vi "Receive Value Change Event.vi"(8 "error in (no error)":errorcluster, 10 "ValueChangeMsg":refnum<class "ValueChangeMsg.lvclass">, 11 "For Loop Dialog In":refnum<class "Conditional Dialog.lvclass">) -> (0 "error out":errorcluster, 3 "For Loop Dialog Out":refnum<class "Conditional Dialog.lvclass">)   [LabVIEW 2017, in "Conditional Dialog.lvclass"]
doc: "<License>\nCopyright © 2017 Composed Systems, LLC | All rights reserved\nwww.composed.io\n\nAuthor: Ethan Stern <ethan.stern@composed.io>\n\nThis software is provided \"AS IS\" WITHOUT WARRANTIES, either express or implied, AND IS FOR EDUCATIONAL PURPOSES ONLY.\n</License>"
uses:
  Conditional Dialog.lvclass
  ITest Executive Builder Dialog/ITest Executive Builder Dialog.lvclass
  <vilib>/gpm_packages/@cs/mva-viewable/Source/ActorEvents/IEventAggregator Messages/ValueChangeMsg/ValueChangeMsg.lvclass
  <vilib>/ActorFramework/Actor/Actor.lvclass
  <vilib>/ActorFramework/Stop Msg/Stop Msg.lvclass
  698eee39-0e44-4932-ada2-d875f71f8c5a.vi
  C:/Program Files (x86)/National Instruments/LabVIEW 2017/vi.lib/ActorFramework/Actor/Actor.lvclass
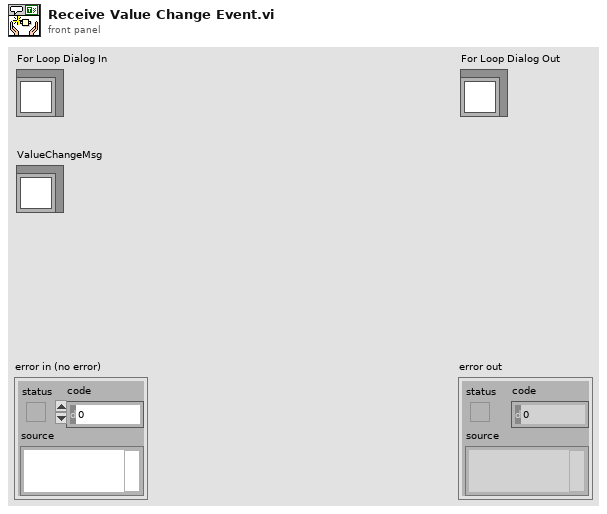
[diagram p1: front panel]
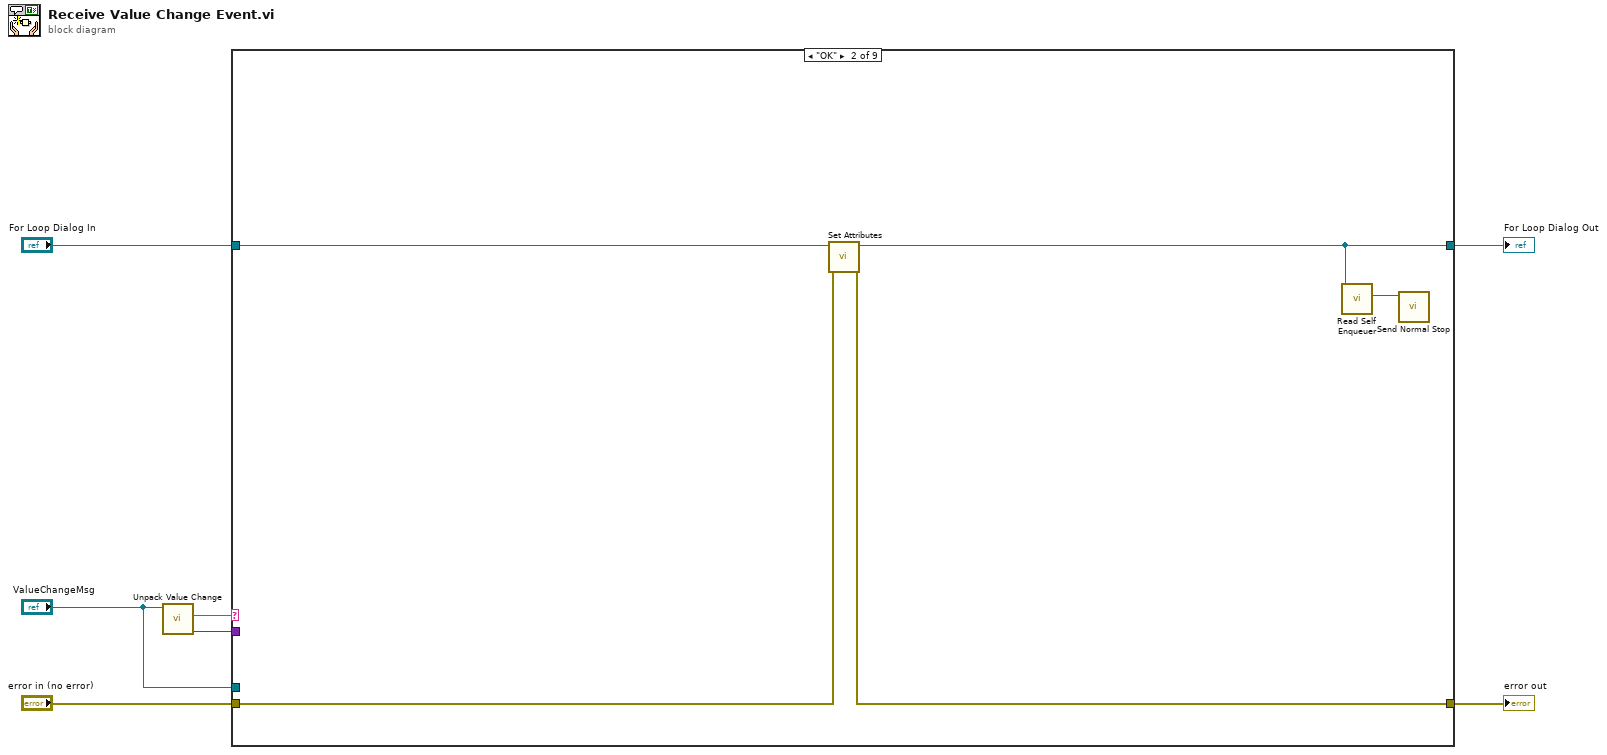
[diagram p0: block diagram]
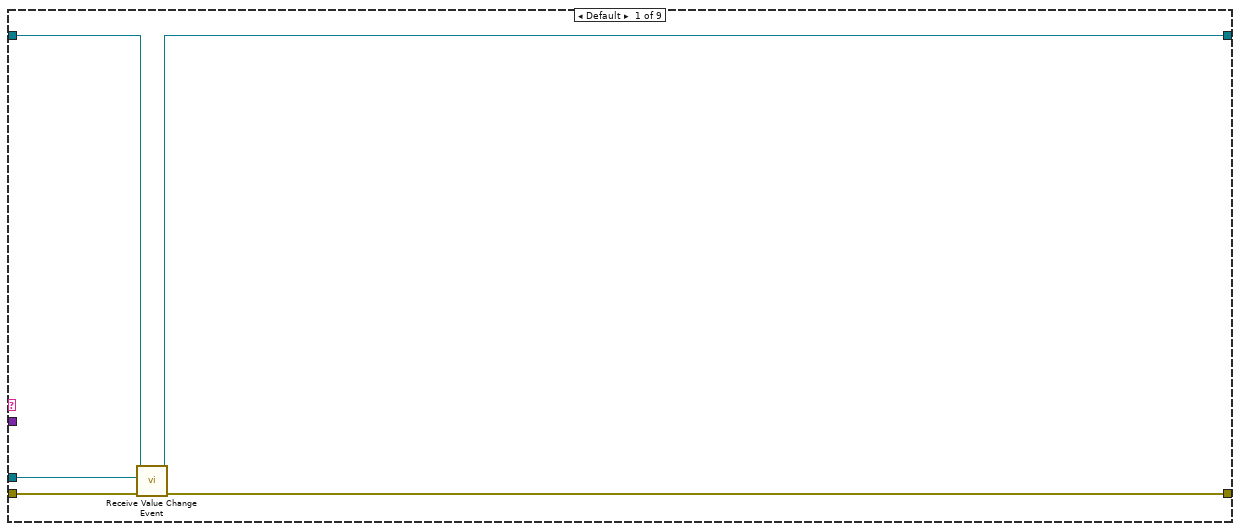
[diagram p2: hidden frame]
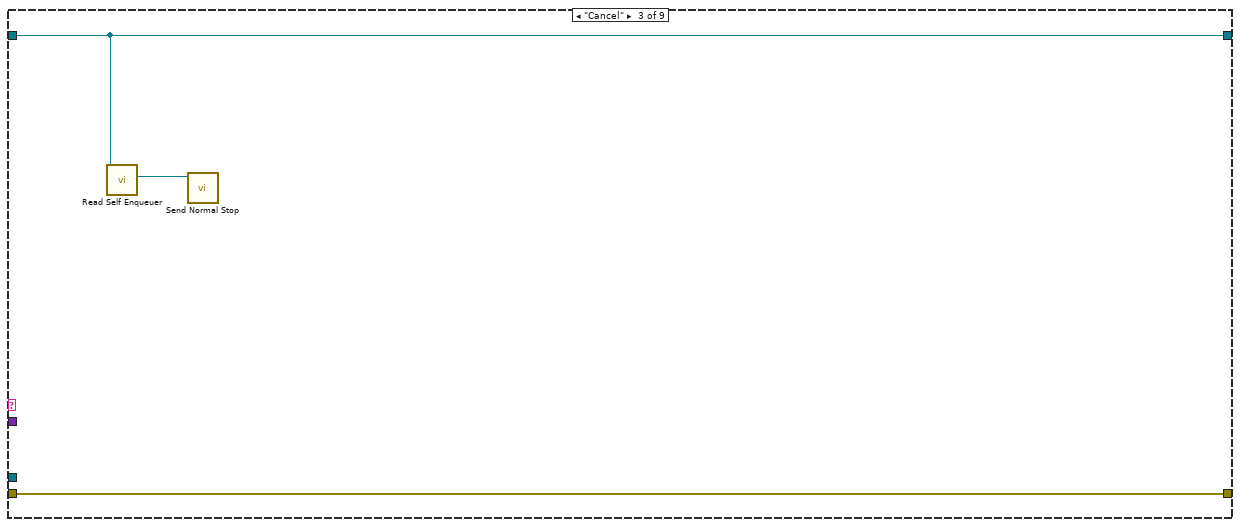
[diagram p3: hidden frame]
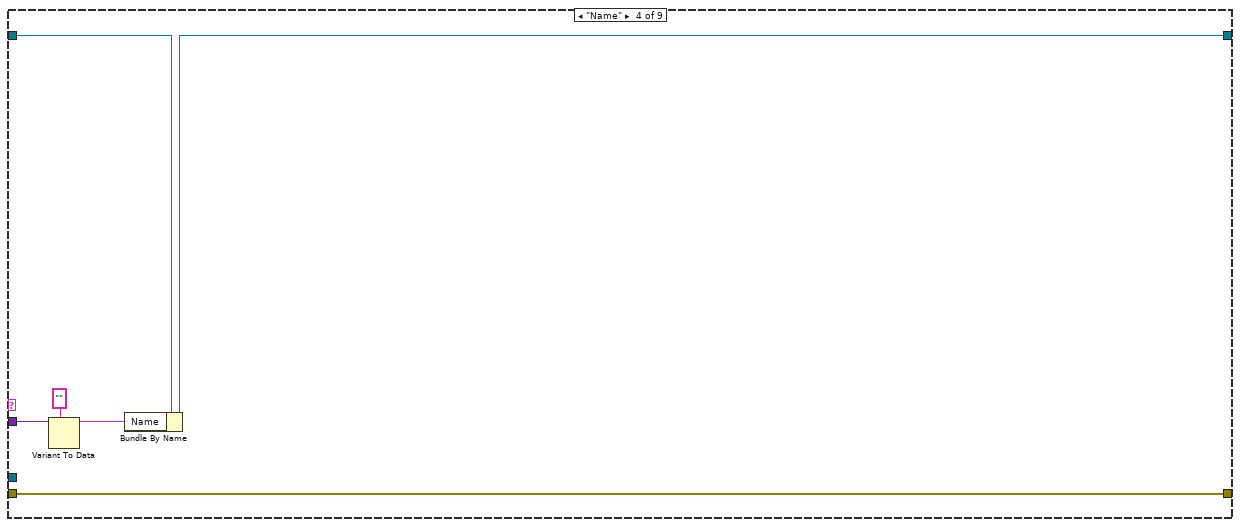
[diagram p4: hidden frame]
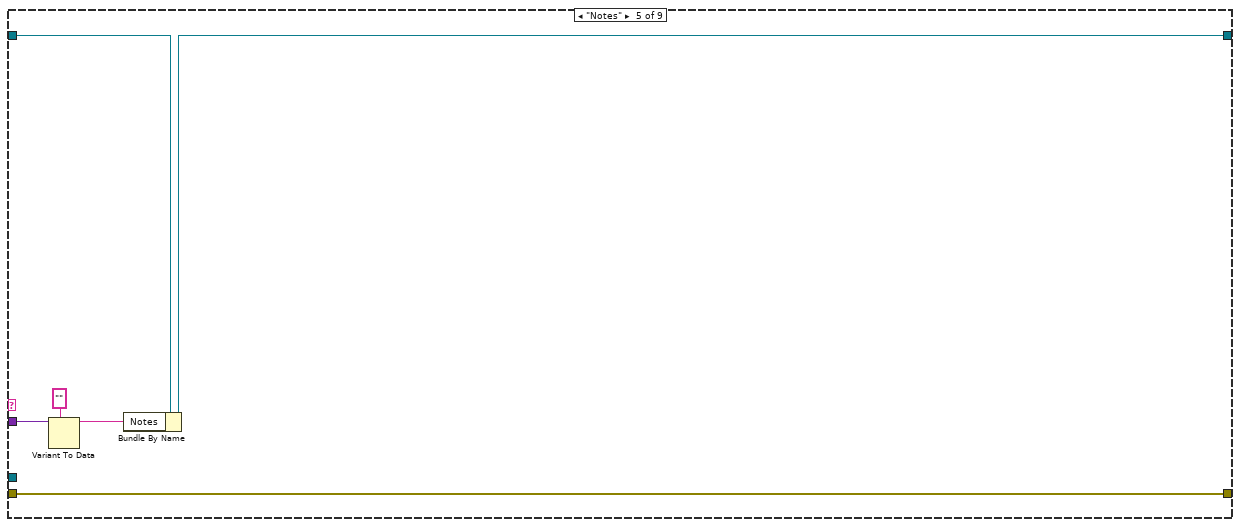
[diagram p5: hidden frame]
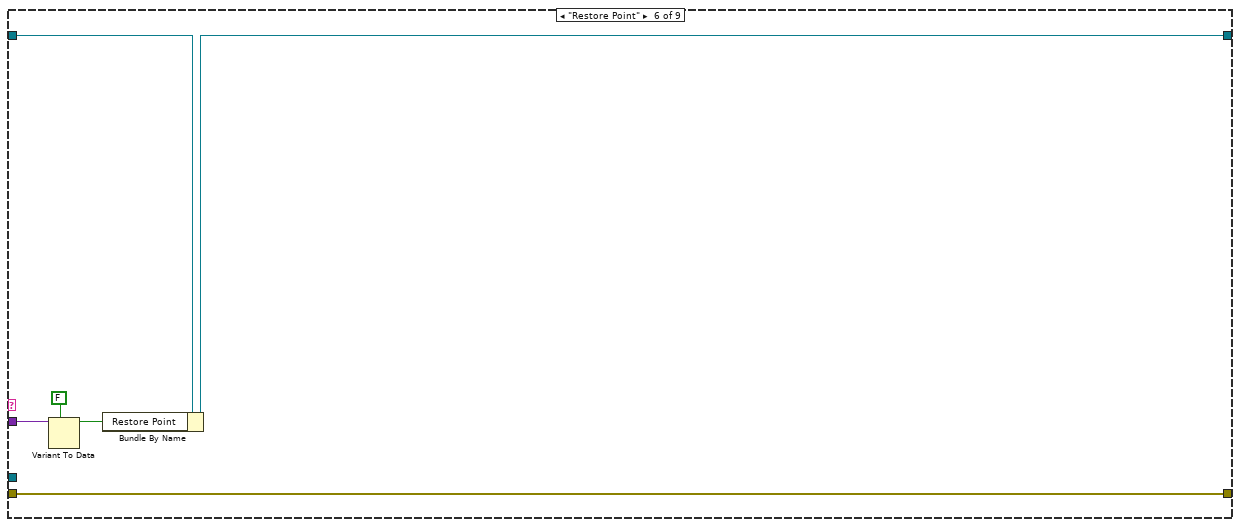
[diagram p6: hidden frame]
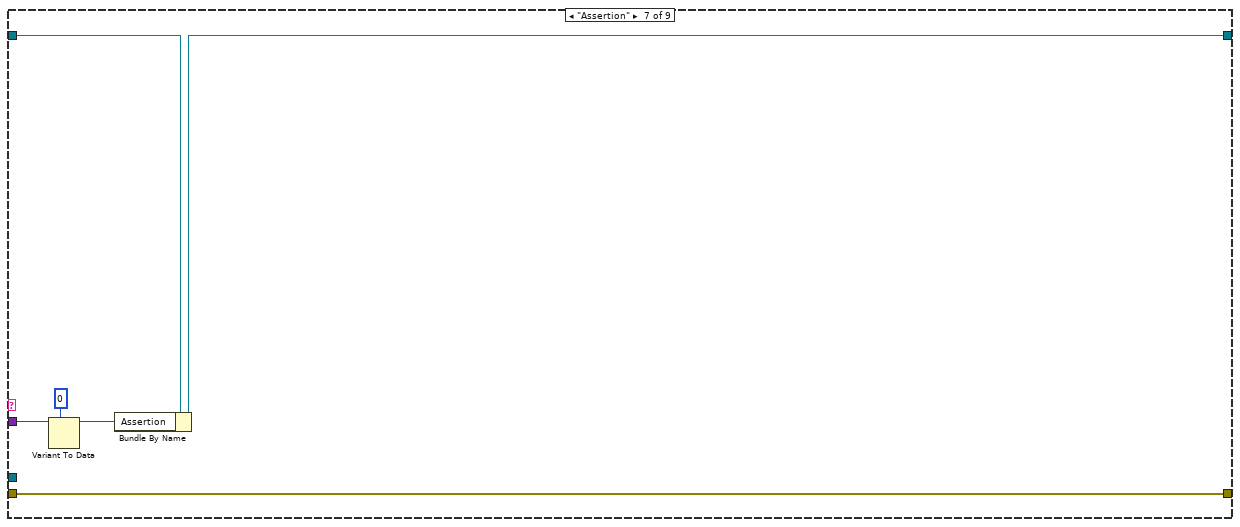
[diagram p7: hidden frame]
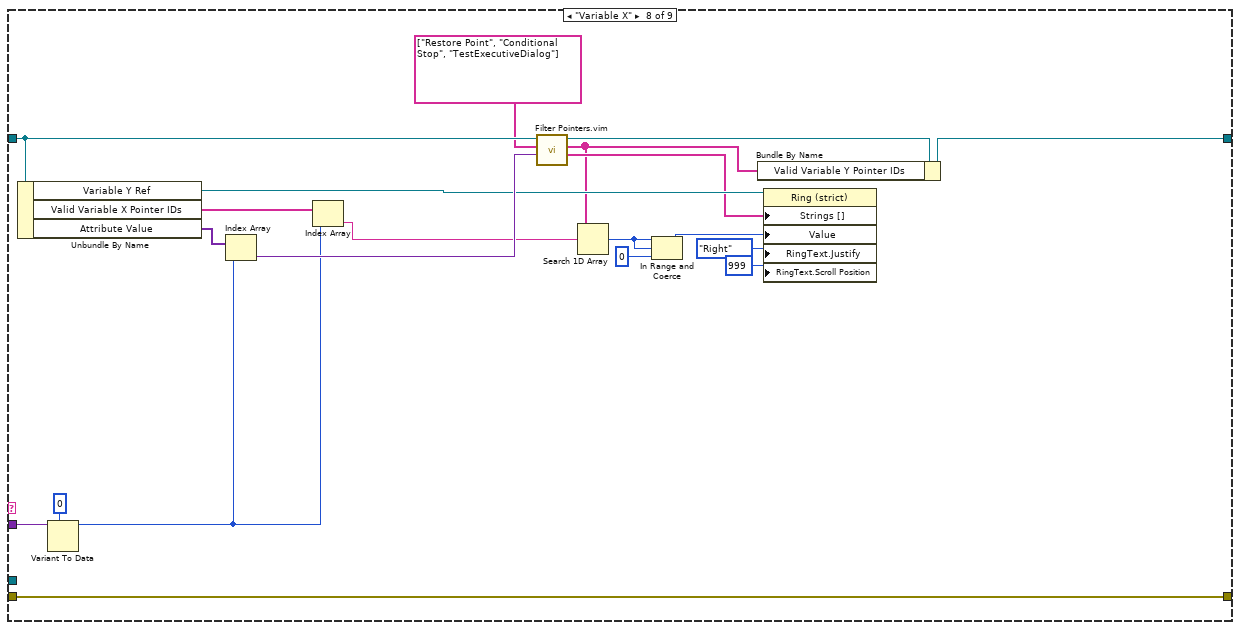
[diagram p8: hidden frame]
diagram:
  n1 = call <vilib>:"Unpack Value Change.vi"("ValueChangeMsg"="ValueChangeMsg") -> ("New Value"=w1:variant, "Control Label"=w2:string)  [unwired: 6 in, 3 out]
  n2 = case shown="\"OK\"" w2 {
    tunnel: [w12 w13 w20 w26 w32 w38 w44 w64 w66] -> w7
    tunnel: [w11 w15 w19 w21 w27 w33 w40 w63 w65] -> w6
    tunnel: "error in (no error)" -> [w10 w14 w20 w26 w32 w38 w44 w64 w66]
    tunnel: "For Loop Dialog In" -> [w9 w16 w19 w22 w28 w34 w41 w62 w65]
    tunnel: "ValueChangeMsg" -> [w8 _ _ _ _ _ _ _ _]
    tunnel: w1 -> [_ _ _ w25 w31 w37 w43 w61 _]
    frame Default {
      n3 = call-parent "Receive Value Change Event.vi"("error in (no error)"=w10, "ValueChangeMsg"=w8, "IViewable In"=w9) -> ("error out"=w12:errorcluster, "IViewable Out"=w11:refnum<class "Conditional Dialog.lvclass">)  [unwired: 7 in]
    }
    frame "OK" {
      n4 = call-dynamic "Set Attributes.vi"("error in (no error)"=w14, "Conditional Dialog in"=w16) -> ("error out"=w13:errorcluster, "Conditional Dialog out"=w15:refnum<class "Conditional Dialog.lvclass">)  [unwired: 8 in]
      n5 = call <vilib>:"Read Self Enqueuer.vi"("Actor"=w15) -> ("Self Enqueuer"=w17:refnum<class "Message Enqueuer.lvclass">)  [unwired: 10 in]
      n6 = call <vilib>:"Send Normal Stop.vi"("Message Enqueuer"=w17) -> ()  [unwired: 10 in, 1 out]
    }
    frame "Cancel" {
      n7 = call <vilib>:"Read Self Enqueuer.vi"("Actor"=w19) -> ("Self Enqueuer"=w18:refnum<class "Message Enqueuer.lvclass">)  [unwired: 10 in]
      n8 = call <vilib>:"Send Normal Stop.vi"("Message Enqueuer"=w18) -> ()  [unwired: 10 in, 1 out]
    }
    frame "Name" {
      n9 = Variant To Data(type="" ("Iterations"), Variant=w25) -> (data=w23:string)  [unwired: 1 in, 1 out]
      n10 = Bundle By Name(cluster=w22, "Name"=w23) -> (w21:refnum<class "Conditional Dialog.lvclass">)
    }
    frame "Notes" {
      n11 = Variant To Data(type="" ("Iterations"), Variant=w31) -> (data=w29:string)  [unwired: 1 in, 1 out]
      n12 = Bundle By Name(cluster=w28, "Notes"=w29) -> (w27:refnum<class "Conditional Dialog.lvclass">)
    }
    frame "Restore Point" {
      n13 = Variant To Data(type=FALSE, Variant=w37) -> (data=w35:bool)  [unwired: 1 in, 1 out]
      n14 = Bundle By Name(cluster=w34, "Restore Point"=w35) -> (w33:refnum<class "Conditional Dialog.lvclass">)
    }
    frame "Assertion" {
      n15 = Variant To Data(type=u16 0 ("Assertion"), Variant=w43) -> (data=w42:u16)  [unwired: 1 in, 1 out]
      n16 = Bundle By Name(cluster=w41, "Assertion"=w42) -> (w40:refnum<class "Conditional Dialog.lvclass">)
    }
    frame "Variable X" {
      n17 = Unbundle By Name(w62) -> ("Variable Y Ref"=w55:refnum<vi>, "Valid Variable X Pointer IDs"=w58:string[], "Attribute Value"=w59:variant[])
      n18 = Variant To Data(type=u16 0, Variant=w61) -> (data=w54:u16)  [unwired: 1 in, 1 out]
      n19 = Index Array(array=w59, index=w54) -> (element=w57:variant)
      n20 = Index Array(array=w58, index=w54) -> (element=w56:string)
      n21 = call "Filter Pointers.vim"("Type"=w57, "Exclusion List"=string[] ["Restore Point", "Conditional Stop", "TestExecutiveDialog"], "ITest Executive Builder Dialog in"=w62) -> ("Valid Pointer Names"=w50:string[], "Valid Pointer IDs"=w48:string[], "ITest Executive Builder Dialog out"=w49:refnum<class "Conditional Dialog.lvclass">)  [unwired: 5 in, 1 out]
      n22 = Search 1D Array(1D array=w48, element=w56) -> (index of element=w47:i32)  [unwired: 1 in]
      n23 = In Range and Coerce(upper limit=w47, x=w47, lower limit=0) -> (coerced(x)=w45:i32)  [unwired: 1 out]
      n24 = Bundle By Name(cluster=w49, "Valid Variable Y Pointer IDs"=w48) -> (w63:refnum<class "Conditional Dialog.lvclass">)
      n25 = property class="Ring (strict)"(reference=w55, "Strings []"=w50, "Value"=w45, "RingText.Justify"=enum16{"Left", "Center", "Right"}."Right" ("Ring Text.Justification"), "RingText.Scroll Position"=u32 999 ("Ring Text.Scroll Position")) -> ()  [unwired: 1 in, 2 out]
    }
    frame "Variable Y" {
    }
  }
  "error out" <- w7
  "For Loop Dialog Out" <- w6
